vi "Seconds_to_hours.vi"() -> ()   [LabVIEW 2015]
panel:
  out "Minutes":i32=60
  out "Hours":i32=60
  out "Seconds":i32=60
  in  "Input Time":i32=60
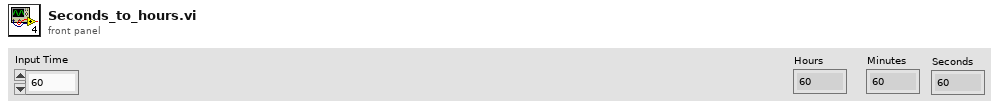
[diagram p1: front panel]
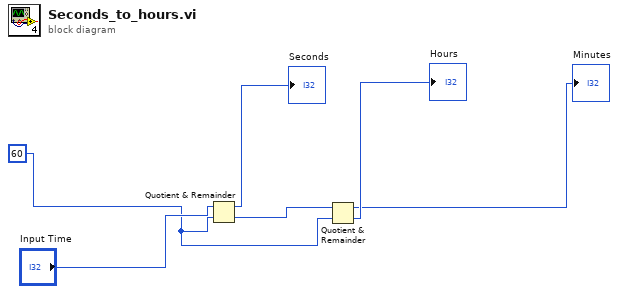
[diagram p0: block diagram]
diagram:
  w1 = 60
  n1 = Quotient & Remainder(x="Input Time", y=w1) -> (x-y*floor(x/y)=→"Seconds":i32, floor(x/y)=w5:i32)
  n2 = Quotient & Remainder(x=w5, y=w1) -> (x-y*floor(x/y)=→"Minutes":i32, floor(x/y)=→"Hours":i32)
